vi "LDT Telescope Get Command ID.vi"() -> (2 "Command ID Str":string, 3 "Command ID":i32)   [LabVIEW 2022 SP3, in "LDT Telescope.lvclass"]
uses:
  LDT Telescope.lvclass
  LDT Telescope.lvclass/LDT Telescope.ctl
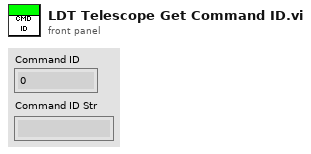
[diagram p1: front panel]
types:
  T1 = typedef "LVDateTimeRec.ctl" = cluster{"fractional second":dbl, "second":i32, "minute":i32, "hour":i32, "day of month":i32, "month":i32, "year":i32, "day of week":i32, "day of year":i32, "DST":i32}
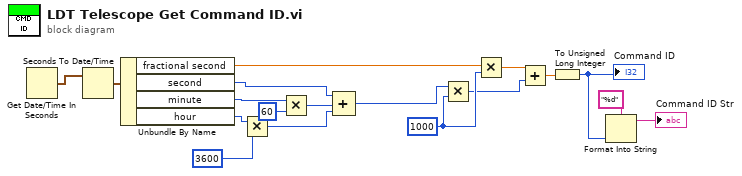
[diagram p0: block diagram]
diagram:
  w15 = 1000 ("y")
  n1 = Get Date/Time In Seconds() -> (seconds since 1Jan1904=w18:timestamp)
  n2 = Seconds To Date/Time(time stamp (now)=w18) -> (date time rec=w17:T1)  [unwired: 1 in]
  n3 = Unbundle By Name(w17) -> ("fractional second"=w16:dbl, "second"=w5:i32, "minute"=w9:i32, "hour"=w11:i32)
  n4 = Multiply(x=w11, y=3600) -> (x*y=w6:i32)
  n5 = Multiply(x=w9, y=60) -> (x*y=w7:i32)
  n6 = Compound Arithmetic op=ADD(w5, w7, w6) -> (w4:i32)
  n7 = Multiply(x=w4, y=w15) -> (x*y=w13:i32)
  n8 = Multiply(x=w16, y=w15) -> (x*y=w14:dbl)
  n9 = Add(x=w14, y=w13) -> (x+y=w12:dbl)
  n10 = To Unsigned Long Integer(number=w12) -> (unsigned 32bit integer=w1:u32)
  "Command ID" <- w1
  n11 = Format Into String(format string="%d", w1) -> (resulting string=→"Command ID Str":string)  [unwired: 2 in, 1 out]
